vi "获取-本机IP地址.vi"(11 "手选?(F)":bool) -> (3 "本机IP":string)   [LabVIEW 2017]
panel:
  in  "本机IP 2":string
  out "IP地址[]":string[](array[string])
  out "MAC地址":string
  out "MAC地址（带分隔符）":string
  out "输出-MAC地址":string caption="标准输出"
  out "输出-IP配置":string caption="标准输出"
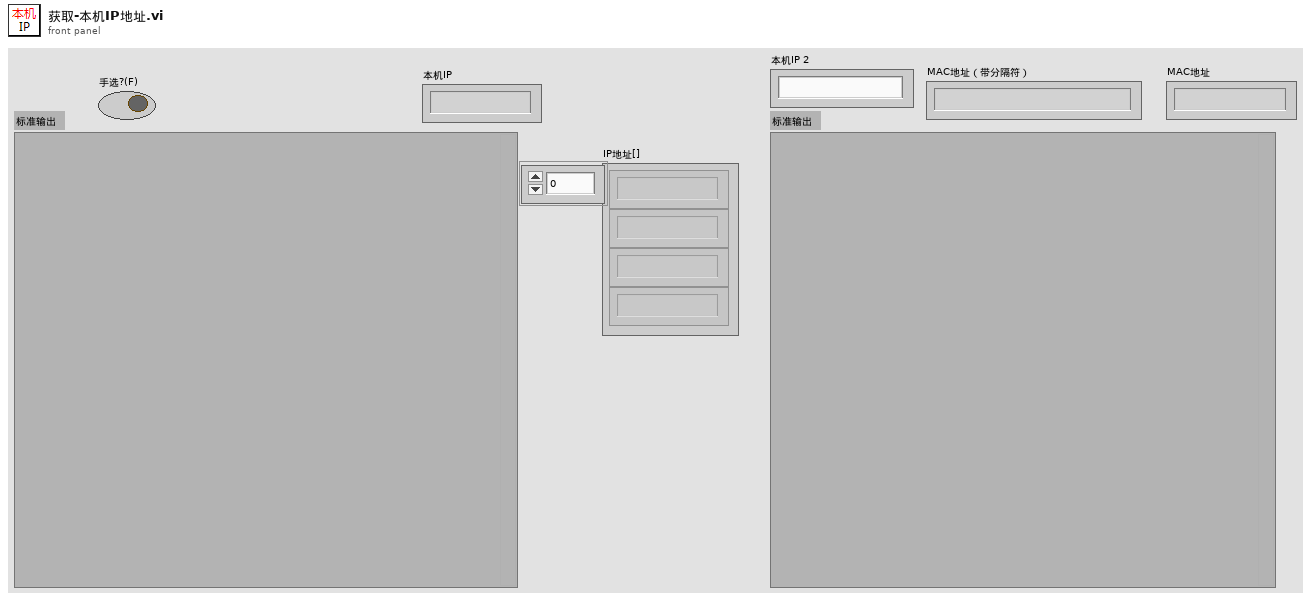
[diagram p1: front panel]
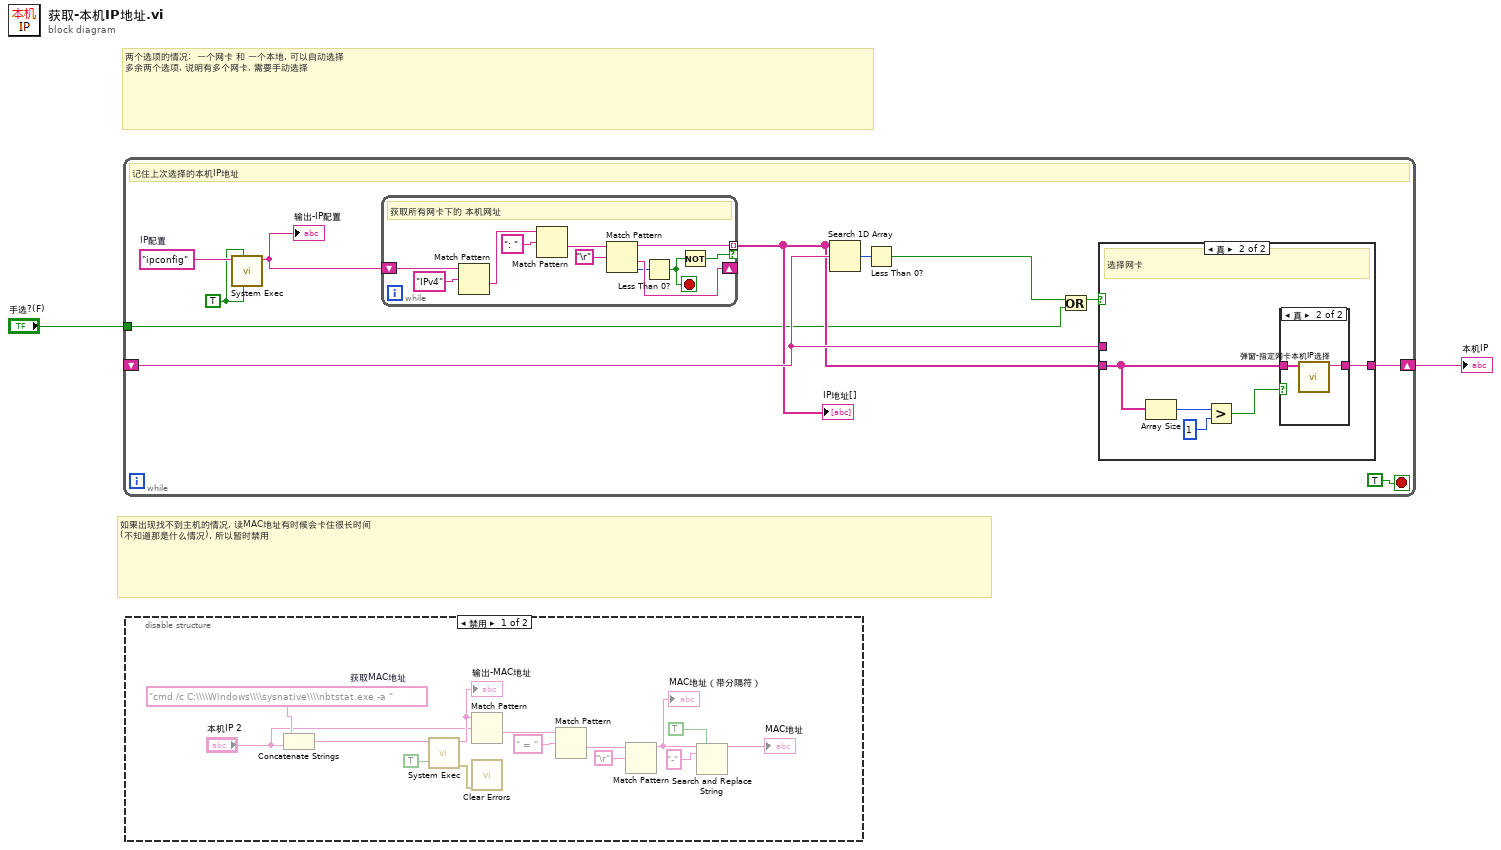
[diagram p0: block diagram]
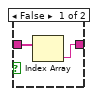
[diagram p3: hidden frame]
diagram:
  # "如果出现找不到主机的情况, 读MAC地址有时候会卡住很长时间\n(不知道那是什么情况), 所以暂时禁用"
  # "两个选项的情况:  一个网卡 和 一个本地, 可以自动选择\n多余两个选项, 说明有多个网卡, 需要手动选择"
  n1 = while {
    shift-right: [w9] -> w2
    shift-left: _ -> [w8]
    tunnel: "手选?(F)" -> [w4]
    stop <- TRUE stop-if-true
    w3 = TRUE ("run minimized? (F)")
    w13 = "ipconfig"  # IP配置
    # "记住上次选择的本机IP地址"
    n2 = call <vilib>:"System Exec.vi"("run minimized? (F)"=w3, "wait until completion? (T)"=w3, "command line"=w13) -> ("standard output"=w6:string)  [unwired: 5 in, 3 out]
    "输出-IP配置" <- w6
    n3 = while {
      shift-right: [w28] -> _
      shift-left: w6 -> [w29]
      tunnel: [w26] -> w7 mode=indexing if=w24
      stop <- w25 stop-if-true
      # "获取所有网卡下的 本机网址"
      n4 = Match Pattern(string=w29, regular expression="IPv4" ("正则表达式")) -> (after substring=w33:string)  [unwired: 1 in, 3 out]
      n5 = Match Pattern(string=w33, regular expression=": " ("正则表达式")) -> (after substring=w31:string)  [unwired: 1 in, 3 out]
      n6 = Match Pattern(string=w31, regular expression="\r") -> (before substring=w26:string, after substring=w28:string, offset past match=w27:i32)  [unwired: 1 in, 1 out]
      n7 = Less Than 0?(x=w27) -> (x < 0?=w25:bool)
      n8 = Not(x=w25) -> (.not. x?=w24:bool)
    }
    "IP地址[]" <- w7
    n9 = Search 1D Array(1D array=w7, element=w8) -> (index of element=w11:i32)  [unwired: 1 in]
    n10 = Less Than 0?(x=w11) -> (x < 0?=w10:bool)
    n11 = Or(x=w10, y=w4) -> (x .or. y?=w5:bool)
    n12 = case shown="真" w5 {
      tunnel: w7 -> [_ w18]
      tunnel: [w14 w19] -> w9
      tunnel: w8 -> [w14 _]
      frame False {
        # "不用选择"
      }
      frame True {
        # "选择网卡"
        n13 = Array Size(array=w18) -> (size(s)=w17:i32)
        n14 = Greater?(x=w17, y=1) -> (0:w15:bool)
        n15 = case shown="真" w15 {
          tunnel: [w20 w23] -> w19
          tunnel: w18 -> [w21 w22]
          frame False {
            n16 = Index Array(array=w21) -> (element=w20:string)  [unwired: 1 in]
          }
          frame True {
            n17 = call "弹窗-指定网卡本机IP选择.vi"("IP地址[]"=w22) -> ("选择的IP"=w23:string)  [unwired: 10 in]
          }
        }
      }
    }
  }
  "本机IP" <- w2
  n18 = disable-structure shown="禁用" {
    frame Disabled {
      w48 = "cmd /c C:\\\\Windows\\\\sysnative\\\\nbtstat.exe -a "  # 获取MAC地址
      n19 = Concatenate Strings(w48, "本机IP 2") -> (w47:string)
      n20 = call <vilib>:"System Exec.vi"("run minimized? (F)"=TRUE, "command line"=w47) -> ("error out"=w36:errorcluster, "standard output"=w45:string)  [unwired: 6 in, 2 out]
      "输出-MAC地址" <- w45
      n21 = Match Pattern(string=w45, regular expression="本机IP 2") -> (after substring=w44:string)  [unwired: 1 in, 3 out]
      n22 = call <vilib>:"Clear Errors.vi"("error in (no error)"=w36) -> ()  [unwired: 5 in, 2 out]
      n23 = Match Pattern(string=w44, regular expression=" = " ("command line")) -> (after substring=w42:string)  [unwired: 1 in, 3 out]
      n24 = Match Pattern(string=w42, regular expression="\r") -> (before substring=w40:string)  [unwired: 1 in, 3 out]
      "MAC地址（带分隔符）" <- w40
      n25 = Search and Replace String(replace all?=TRUE ("替换全部？(F)"), input string=w40, search string="-" ("搜索字符串")) -> (result string=→"MAC地址":string)  [unwired: 5 in, 3 out]
    }
    frame Enabled {
    }
  }
